vi "ex_userDefPropDialog.vi"(9 "Configure User Def Prop Control":T4(xcontrol)) -> (1 "Data Out":T4(xcontrol), 2 "Cancelled?":bool)   [LabVIEW 2020]
uses:
  <vilib>/Platform/express/ex_EditUserDefinedProperties/Configure User Def Prop.xctl
panel:
  in  "Help":bool
  in  "Cancel":bool
  in  "OK":bool
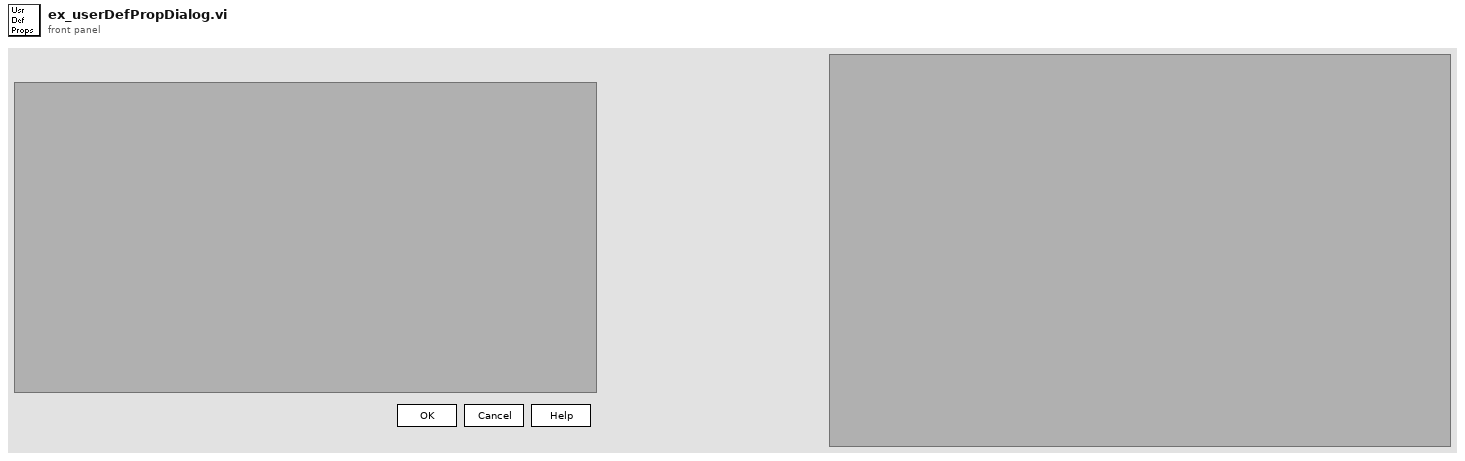
[diagram p1: front panel]
types:
  T1 = typedef "ex_userDefProperty.ctl" = cluster{"Name":string, "Object type":string, "usiDataType":T2, "propertySourceType":T3, "propertySource":string, "Value":variant, "ID":i32, "use def name":bool, "Source":string, "Built-in Prop":bool, "Attribute Type Enum":string[]}
  T2 = typedef "usiDataType.ctl" = enum16{"eNoTypeUsi", "eInt8Usi", "eInt16Usi", "eInt32Usi", "eInt64Usi", "eUInt8Usi", "eUInt16Usi", "eUInt32Usi", "eUInt64Usi", "eFloat32Usi", "eFloat64Usi", "- 0", "- 1", "- 2", "- 3", "- 4", "- 5", "- 6", "- 7", "- 8", "- 9", "eString8Usi", "eString16Usi", "eStringUsi", "eEnumUsi", "- 10", "- 11", "- 12", "- 13", "- 14", "eTimeUsi", "- 15", "- 16", "- 17", "- 18", "- 19", "- 20", "- 21", "- 22", "- 23", "eInstanceUsi", "eStoreUsi"}
  T3 = typedef "ex_propertySource.ctl" = enum16{"Manual", "System", "DAQmx Channel", "Terminal", "Ignore"}
  T4 = cluster{"user-def properties in":T1[], "selected nodes in":string[]}
  T5 = cluster{"CallerInfo":cluster{"Caller Type":enum16{"default", "storage write", "storage read", "measurement write"}, "Object Type":string}}
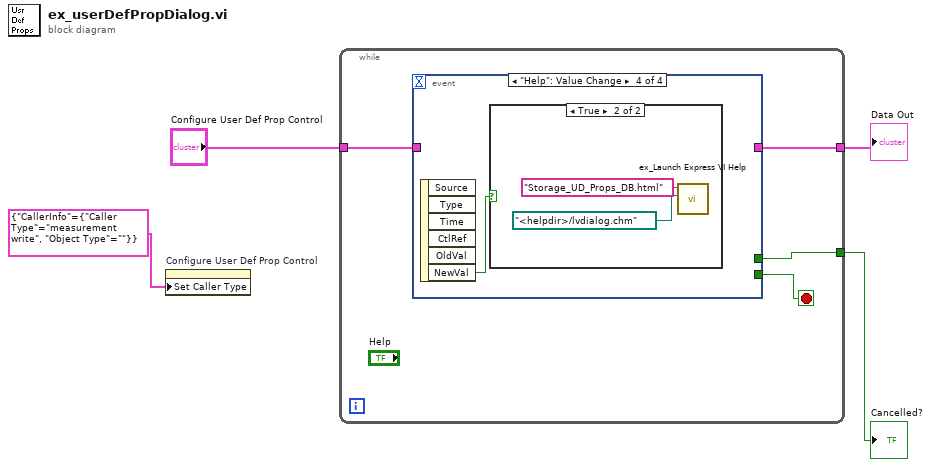
[diagram p0: block diagram]
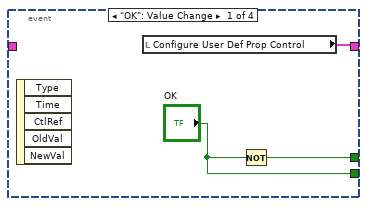
[diagram p2: hidden frame]
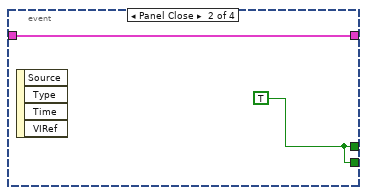
[diagram p3: hidden frame]
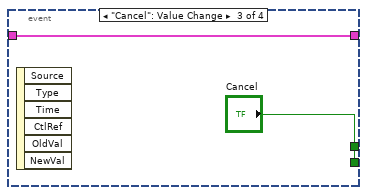
[diagram p4: hidden frame]
diagram:
  n1 = property on="Configure User Def Prop Control" class="Configure User Def Prop (strict"("Set Caller Type"=T5 {"CallerInfo"={"Caller Type"=enum."measurement write", "Object Type"=""}}) -> ()  [unwired: 2 in, 2 out]
  n2 = while {
    tunnel: [w7] -> w2
    tunnel: "Configure User Def Prop Control" -> [w6]
    tunnel: [w5] -> w4
    stop <- w8 stop-if-true
    n3 = event shown="[3] \"Help\": Value Change" {
      selector: _ -> [_ _ _ _]
      dyn-events: _ -> [_ _ _ _]
      timeout: _ -> [_ _ _ _]
      tunnel: ["OK" w12 "Cancel" _] -> w8
      tunnel: [w10 w12 "Cancel" _] -> w7
      tunnel: [w9 w13 w14 _] -> w5
      tunnel: w6 -> [_ w13 w14 _]
      event "OK": Value Change {
        n4 = event-data() -> ()  [unwired: 6 out]
        n5 = local read "Configure User Def Prop Control"() -> (w9:T4)
        n6 = Not(x="OK") -> (.not. x?=w10:bool)
      }
      event Panel Close {
        w12 = TRUE
        n7 = event-data() -> ()  [unwired: 5 out]
      }
      event "Cancel": Value Change {
        n8 = event-data() -> ()  [unwired: 7 out]
      }
      event "Help": Value Change {
        n9 = event-data() -> ("NewVal"=w16:bool)  [unwired: 6 out]
        n10 = case shown="True" w16 {
          frame False {
          }
          frame True {
            n11 = call <vilib>:"ex_Launch Express VI Help.vi"("Help File Path"=path "<helpdir>/lvdialog.chm", "Keyword/HTML File"="Storage_UD_Props_DB.html") -> ()  [unwired: 1 in, 5 out]
          }
        }
      }
    }
  }
  "Cancelled?" <- w2
  "Data Out" <- w4
